vi "Melt-pool-characteristics.vi"(7 "Config. params. ref. in":refnum<data-value>, 8 "error in":errorcluster, 10 "Buffer element in":T1 {"Temperature characteristics"."Stand. dev. temperature" format="%#.1f"; "Temperature characteristics"."Min. temperature" format="%#.0f"; "Temperature characteristics"."Max. temperature" format="%#.0f"; "Temperature characteristics"."Average temperature" format="%#.0f"}, 11 "Analysis params. ref. in":refnum<data-value>) -> (0 "error IO":errorcluster, 2 "Buffer element":T1 {"Temperature characteristics"."Stand. dev. temperature" format="%#.1f"; "Temperature characteristics"."Min. temperature" format="%#.0f"; "Temperature characteristics"."Max. temperature" format="%#.0f"; "Temperature characteristics"."Average temperature" format="%#.0f"}, 3 "Analysis params. ref.":refnum<data-value>, 5 "Config. params. ref.":refnum<data-value>)   [LabVIEW 2013, in "CameraVision.lvlib" / "CV-Main.lvclass"]
uses:
  CV-Main.lvclass
  Configuration/CV-Configuration.lvclass
  Analysis/CV-Analysis.lvclass
  Buffers/Storage-buffer.ctl
  <vilib>/vision/Image Controls.llb/IMAQ Image.ctl
  Temperature/Temperature-characteristics.ctl
  Analysis/Characteristics-cluster.ctl
  Configuration/CV-Configuration.lvclass/CV-Configuration.ctl
  Analysis/CV-Analysis.lvclass/CV-Analysis.ctl
  Analysis/Read Melt-pool connectivity.vi
  Analysis/Read Melt-pool characteristic defaults.vi
  Analysis/Read Melt-pool characteristics.vi
  Configuration/Read Width scale.vi
  Configuration/Read Height scale.vi
  <vilib>/vision/NI_Vision_Development_Module.lvlib
  Temperature/CV-Temperature.lvclass
  Buffers/CV-Buffers.lvclass
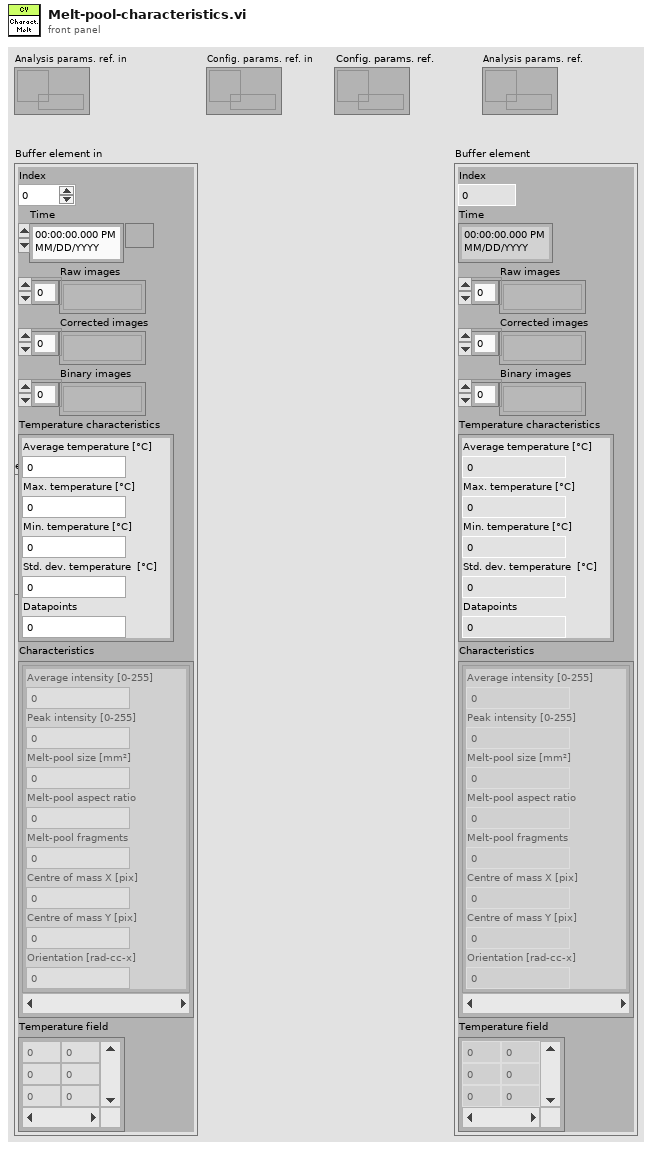
[diagram p1: front panel]
types:
  T1 = typedef "CameraVision.lvlib/CV-Buffers.lvclass/Storage-buffer.ctl" = cluster{"Index":i32, "Time":timestamp, "Raw images":T2[], "Corrected images":T2[], "Binary images":T2[], "Temperature characteristics":T3, "Characteristics":T4[], "Temperature field":dbl[][]}
  T2 = typedef "IMAQ Image.ctl" = refnum<image>
  T3 = typedef "CameraVision.lvlib/CV-Temperature.lvclass/Temperature-characteristics.ctl" = cluster{"Average temperature ":dbl, "Max. temperature":dbl, "Min. temperature":dbl, "Stand. dev. temperature":dbl, "Datapoints":dbl}
  T4 = typedef "CameraVision.lvlib/CV-Analysis.lvclass/Characteristics-cluster.ctl" = cluster{"Average intensity":dbl, "Peak intensity":dbl, "Melt-pool size":dbl, "Melt-pool aspect ratio":dbl, "Melt-pool fragments":dbl, "Centre of mass X":dbl, "Centre of mass Y":dbl, "Orientation":dbl}
  T5 = typedef "Particle Parameters" = i32
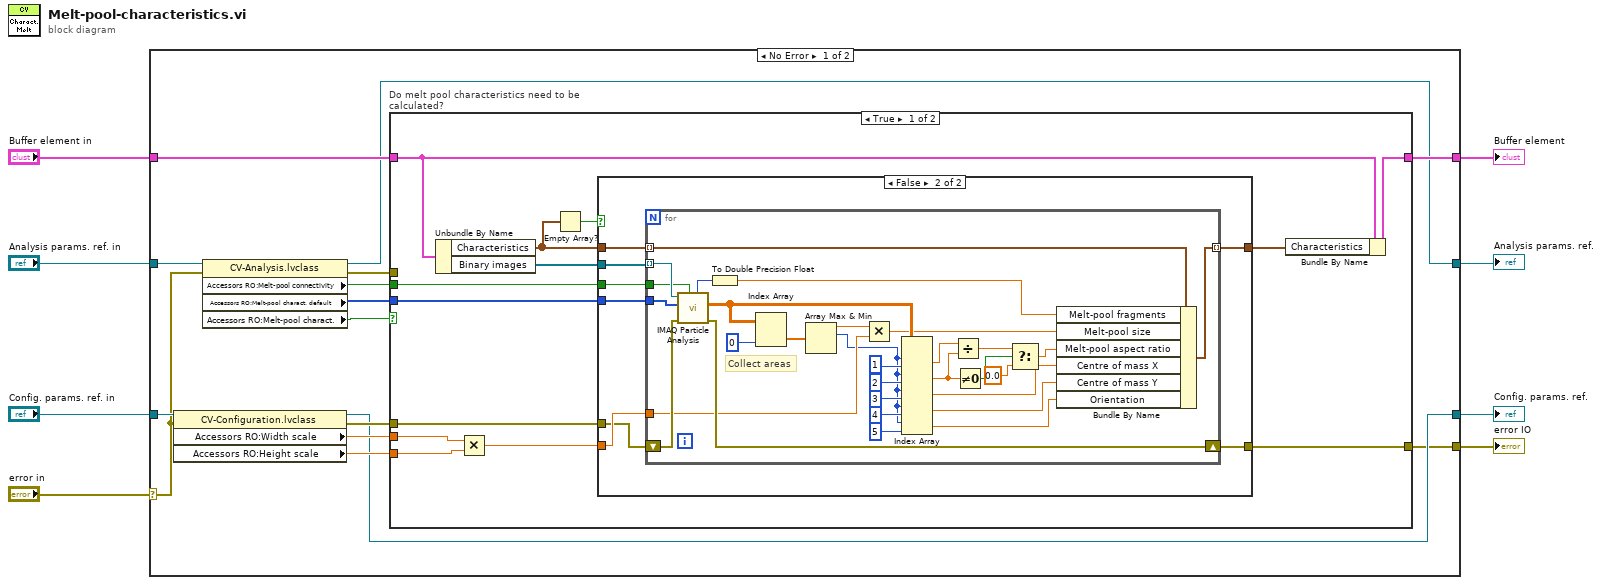
[diagram p0: block diagram]
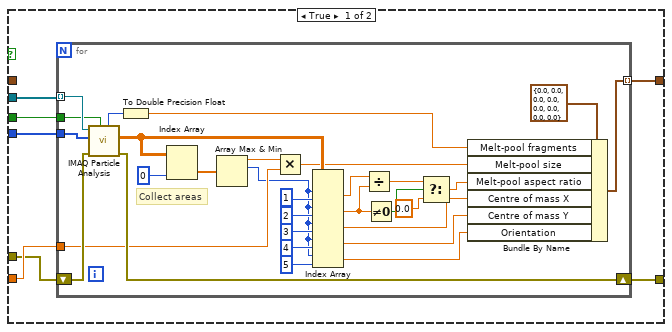
[diagram p2: hidden frame]
diagram:
  n1 = case shown="No Error" "error in" {
    selector: "error in" -> [w15 w117]
    tunnel: [w9 w117] -> w7
    tunnel: "Buffer element in" -> [w12 w115]
    tunnel: "Config. params. ref. in" -> [w19 w114]
    tunnel: "Analysis params. ref. in" -> [w23 w116]
    tunnel: [w10 w116] -> w3
    tunnel: [w11 w115] -> w2
    tunnel: [w13 w114] -> w1
    frame No Error {
      n2 = property class="CV-Configuration.lvclass"(reference=w19, error in=w15) -> (reference out=w13:refnum<data-value>, error out=w14:errorcluster, "Accessors RO:Width scale"=w18:dbl, "Accessors RO:Height scale"=w17:dbl)
      n3 = property class="CV-Analysis.lvclass"(reference=w23, error in=w15) -> (reference out=w10:refnum<data-value>, error out=w16:errorcluster, "Accessors RO:Melt-pool connectivity"=w22:bool, "Accessors RO:Melt-pool charact. default"=w21:T5[], "Accessors RO:Melt-pool charact."=w20:bool)
      n4 = case "Do melt pool characteristics need to be calculated?" shown="True" w20 {
        tunnel: w12 -> [w29 w112]
        tunnel: [w31 w113] -> w9
        tunnel: w18 -> [w36 _]
        tunnel: w17 -> [w35 _]
        tunnel: w22 -> [w33 _]
        tunnel: w21 -> [w30 _]
        tunnel: w16 -> [_ _]
        tunnel: w14 -> [w32 w113]
        tunnel: [w25 w112] -> w11
        frame True {
          n5 = Unbundle By Name(w29) -> ("Characteristics"=w27:T4[], "Binary images"=w26:T2[])
          n6 = Multiply(x=w36, y=w35) -> (x*y=w34:dbl)
          n7 = Empty Array?(array=w27) -> (empty?=w28:bool)
          n8 = case shown="False" w28 {
            tunnel: w34 -> [w43 w81]
            tunnel: w33 -> [w42 w80]
            tunnel: w32 -> [w41 w79]
            tunnel: [w40 w78] -> w31
            tunnel: [w39 w77] -> w24
            tunnel: w30 -> [w38 w76]
            tunnel: w27 -> [_ w74]
            tunnel: w26 -> [w37 w75]
            frame True {
              n9 = for {
                tunnel: w37 -> [w73] mode=indexing
                tunnel: w38 -> [w72]
                shift-right: [w64] -> w40
                shift-left: w41 -> [w65]
                tunnel: w43 -> [w61]
                tunnel: [w56] -> w39 mode=indexing
                tunnel: w42 -> [w57]
                # "Collect areas"
                n10 = call "IMAQ Particle Analysis"("Connectivity 4/8 (8)"=w57, "error in (no error)"=w65, "Pixel Measurements"=w72, "Image"=w73) -> ("error out"=w64:errorcluster, "Particle Measurements (Pixels)"=w68:dbl[][], "Number of Particles"=w71:i32)  [unwired: 2 in, 3 out]
                n11 = To Double Precision Float(number=w71) -> (double precision float=w66:dbl)
                n12 = Index Array(array=w68, index (col)=0 ("disabled index (col)")) -> (element=w69:dbl[])  [unwired: 1 in]
                n13 = Array Max & Min(array=w69) -> (max value=w62:dbl, max index (indices)=w53:i32)  [unwired: 2 out]
                n14 = Multiply(x=w62, y=w61) -> (x*y=w63:dbl)
                n15 = Index Array(array=w68, index (row) #1=w53, index (col) #1=1 ("disabled index (col)"), index (row) #2=w53, index (col) #2=2 ("disabled index (col)"), index (row) #3=w53, index (col) #3=3 ("disabled index (col)"), index (row) #4=w53, index (col) #4=4 ("disabled index (col)"), index (row) #5=w53, index (col) #5=5 ("index (col)")) -> (element #1=w55:dbl, element #2=w49:dbl, element #3=w52:dbl, element #4=w51:dbl, element #5=w50:dbl)
                n16 = Divide(x=w55, y=w49) -> (x/y=w47:dbl)
                n17 = Not Equal To 0?(x=w49) -> (x != 0?=w48:bool)
                n18 = Select(t=w47, s=w48, f=0.0) -> (s? t:f=w46:dbl)
                n19 = Bundle By Name(cluster=T4 {"Average intensity"=0.0, "Peak intensity"=0.0, "Melt-pool size"=0.0, "Melt-pool aspect ratio"=0.0, "Melt-pool fragments"=0.0, "Centre of mass X"=0.0, "Centre of mass Y"=0.0, "Orientation"=0.0} ("Characteristics"), "Melt-pool fragments"=w66, "Melt-pool size"=w63, "Melt-pool aspect ratio"=w46, "Centre of mass X"=w52, "Centre of mass Y"=w51, "Orientation"=w50) -> (w56:T4)
              }
            }
            frame False {
              n20 = for {
                tunnel: w75 -> [w111] mode=indexing
                tunnel: w76 -> [w110]
                shift-right: [w102] -> w78
                shift-left: w79 -> [w103]
                tunnel: w81 -> [w99]
                tunnel: [w94] -> w77 mode=indexing
                tunnel: w80 -> [w95]
                tunnel: w74 -> [w82] mode=indexing
                # "Collect areas"
                n21 = call "IMAQ Particle Analysis"("Connectivity 4/8 (8)"=w95, "error in (no error)"=w103, "Pixel Measurements"=w110, "Image"=w111) -> ("error out"=w102:errorcluster, "Particle Measurements (Pixels)"=w106:dbl[][], "Number of Particles"=w109:i32)  [unwired: 2 in, 3 out]
                n22 = To Double Precision Float(number=w109) -> (double precision float=w104:dbl)
                n23 = Index Array(array=w106, index (col)=0 ("disabled index (col)")) -> (element=w107:dbl[])  [unwired: 1 in]
                n24 = Array Max & Min(array=w107) -> (max value=w100:dbl, max index (indices)=w91:i32)  [unwired: 2 out]
                n25 = Multiply(x=w100, y=w99) -> (x*y=w101:dbl)
                n26 = Index Array(array=w106, index (row) #1=w91, index (col) #1=1 ("disabled index (col)"), index (row) #2=w91, index (col) #2=2 ("disabled index (col)"), index (row) #3=w91, index (col) #3=3 ("disabled index (col)"), index (row) #4=w91, index (col) #4=4 ("disabled index (col)"), index (row) #5=w91, index (col) #5=5 ("index (col)")) -> (element #1=w93:dbl, element #2=w87:dbl, element #3=w90:dbl, element #4=w89:dbl, element #5=w88:dbl)
                n27 = Divide(x=w93, y=w87) -> (x/y=w85:dbl)
                n28 = Not Equal To 0?(x=w87) -> (x != 0?=w86:bool)
                n29 = Select(t=w85, s=w86, f=0.0) -> (s? t:f=w84:dbl)
                n30 = Bundle By Name(cluster=w82, "Melt-pool fragments"=w104, "Melt-pool size"=w101, "Melt-pool aspect ratio"=w84, "Centre of mass X"=w90, "Centre of mass Y"=w89, "Orientation"=w88) -> (w94:T4)
              }
            }
          }
          n31 = Bundle By Name(cluster=w29, "Characteristics"=w24) -> (w25:T1)
        }
        frame False {
        }
      }
    }
    frame Error {
    }
  }
  "error IO" <- w7
  "Buffer element" <- w2
  "Analysis params. ref." <- w3
  "Config. params. ref." <- w1
